vi "average_expSD.vi"(1 "Experiments groups":refnum<class "Experiments_group.lvclass">[](array[class]), 2 "group":u16) -> (0 "averaged data":dbl[][](array[numeric]))   [LabVIEW 2015]
uses:
  Classes/Experiment.lvclass
  Classes/Experiments_group.lvclass
panel:
  in  "error in (no error)":errorcluster
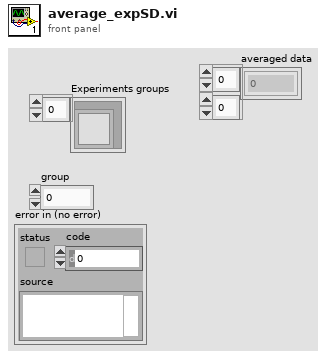
[diagram p1: front panel]
types:
  T1 = cluster{"Lower limit W":dbl, "Upper limit W":dbl}
  T2 = cluster{"Lower limit TD":dbl, "Upper limit TD":dbl}
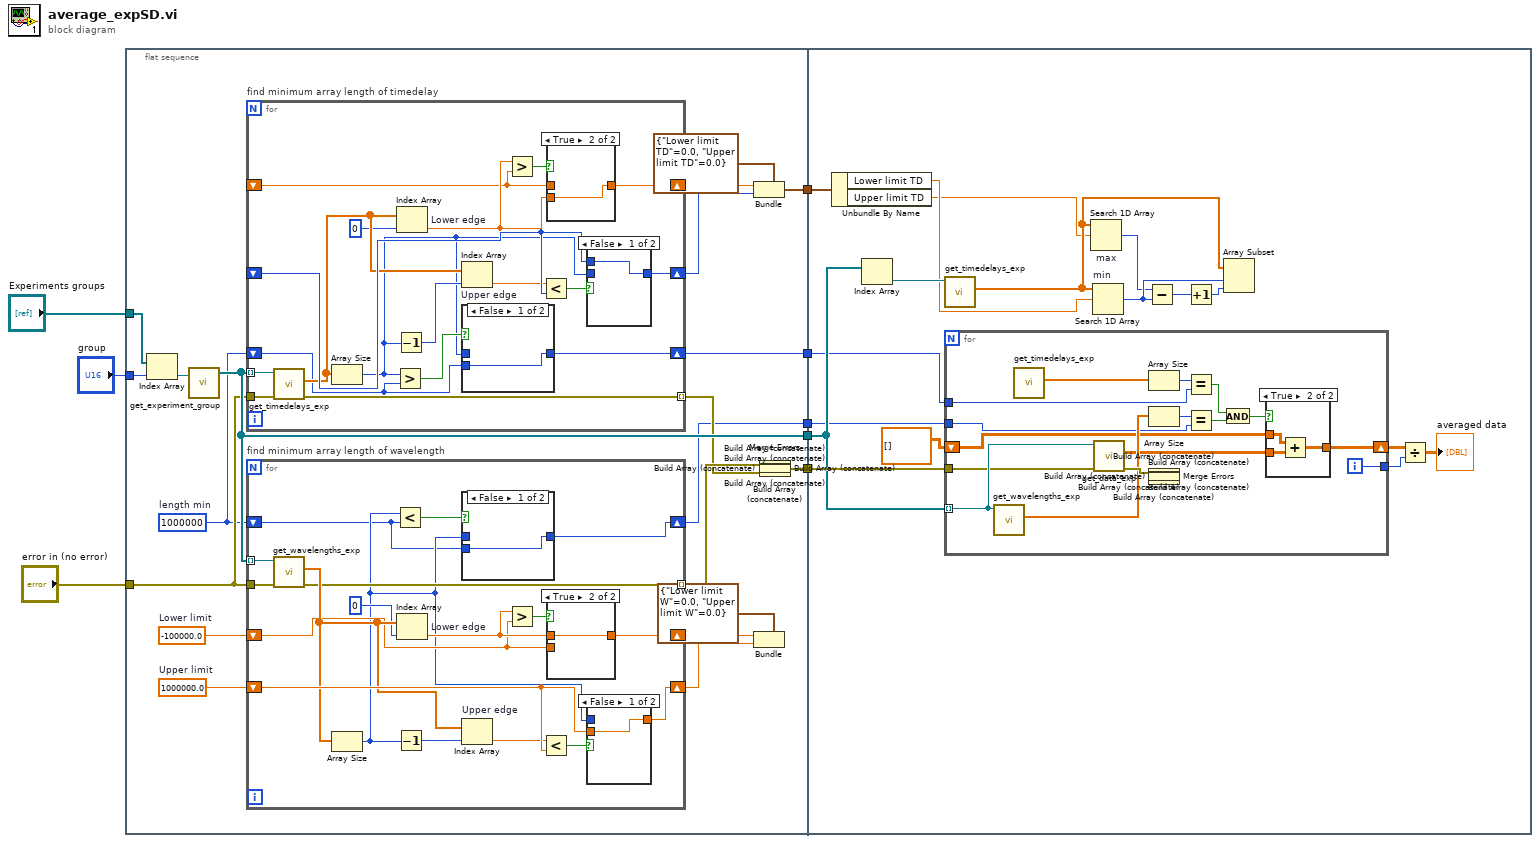
[diagram p0: block diagram]
diagram:
  n1 = flat-sequence {
    tunnel: "group" -> [w33]
    tunnel: "Experiments groups" -> [w32]
    tunnel: "error in (no error)" -> [w19]
    tunnel: [w23] -> w5
    tunnel: [w20] -> w4
    tunnel: [w18] -> w3
    tunnel: [w16] -> w2
    tunnel: [w15] -> w1
    tunnel: w5 -> [w88]
    tunnel: w4 -> [w95]
    tunnel: w3 -> [w94]
    tunnel: w2 -> [w84]
    tunnel: w1 -> [w83]
    frame #0 {
      w17 = 1000000  # length min
      w30 = -100000.0  # Lower limit
      w31 = 1000000.0  # Upper limit
      n2 = Index Array(array=w32, index=w33) -> (element=w34:refnum<class "Experiments_group.lvclass">)
      n3 = call-dynamic "get_experiment_group.vi"("Experiments_group.lvclass in"=w34) -> ("Experiments"=w23:refnum<class "Experiment.lvclass">[])  [unwired: 1 in, 2 out]
      n4 = for "find minimum array length of timedelay" {
        tunnel: w23 -> [w52] mode=indexing
        tunnel: w19 -> [w51]
        shift-right: [w49] -> w25
        shift-left: _ -> [w48]
        shift-right: [w42] -> w24
        shift-left: _ -> [w41]
        tunnel: [w39] -> w21 mode=indexing
        shift-right: [w37] -> w15
        shift-left: w17 -> [w35]
        n5 = call-dynamic "get_timedelays_exp.vi"("error in (no error)"=w51, "Experiment.lvclass in"=w52) -> ("error out"=w39:errorcluster, "timedelays"=w45:dbl[])  [unwired: 7 in, 1 out]
        n6 = Array Size(array=w45) -> (size(s)=w36:i32)
        n7 = Greater?(x=w36, y=w35) -> (0:w38:bool)
        n8 = Decrement(x=w36) -> (x-1=w47:i32)
        n9 = Index Array "Lower edge"(array=w45, index=0) -> (element=w43:dbl)
        n10 = Index Array "Upper edge"(array=w45, index=w47) -> (element=w46:dbl)
        n11 = case shown="False" w38 {
          tunnel: [w53 w54] -> w37
          tunnel: w36 -> [_ w54]
          tunnel: w35 -> [w53 _]
          frame False {
          }
          frame True {
          }
        }
        n12 = Greater?(x=w43, y=w41) -> (0:w40:bool)
        n13 = Less?(x=w46, y=w48) -> (x < y?=w50:bool)
        n14 = case shown="True" w40 {
          tunnel: [w55 w56] -> w42
          tunnel: w43 -> [_ w56]
          tunnel: w41 -> [w55 _]
          frame False {
          }
          frame True {
          }
        }
        n15 = case shown="False" w50 {
          tunnel: [w57 w58] -> w49
          tunnel: w36 -> [_ w58]
          tunnel: w48 -> [w57 _]
          frame False {
          }
          frame True {
          }
        }
      }
      n16 = for "find minimum array length of wavelength" {
        tunnel: w23 -> [w76] mode=indexing
        tunnel: w19 -> [w75]
        shift-right: [w73] -> w28
        shift-left: w31 -> [w72]
        shift-right: [w66] -> w29
        shift-left: w30 -> [w65]
        tunnel: [w63] -> w22 mode=indexing
        shift-right: [w60] -> w16
        shift-left: w17 -> [w59]
        n17 = call-dynamic "get_wavelengths_exp.vi"("error in (no error)"=w75, "Experiment.lvclass in"=w76) -> ("error out"=w63:errorcluster, "wavelengths"=w69:dbl[])  [unwired: 7 in, 1 out]
        n18 = Array Size(array=w69) -> (size(s)=w61:i32)
        n19 = Less?(x=w61, y=w59) -> (x < y?=w62:bool)
        n20 = Decrement(x=w61) -> (x-1=w71:i32)
        n21 = Index Array "Lower edge"(array=w69, index=0) -> (element=w67:dbl)
        n22 = case shown="False" w62 {
          tunnel: w61 -> [_ w78]
          tunnel: [w77 w78] -> w60
          tunnel: w59 -> [w77 _]
          frame False {
          }
          frame True {
          }
        }
        n23 = Index Array "Upper edge"(array=w69, index=w71) -> (element=w70:dbl)
        n24 = Greater?(x=w67, y=w65) -> (0:w64:bool)
        n25 = Less?(x=w70, y=w72) -> (x < y?=w74:bool)
        n26 = case shown="True" w64 {
          tunnel: [w79 w80] -> w66
          tunnel: w67 -> [_ w80]
          tunnel: w65 -> [w79 _]
          frame False {
          }
          frame True {
          }
        }
        n27 = case shown="False" w74 {
          tunnel: [w81 w82] -> w73
          tunnel: w61 -> [_ w82]
          tunnel: w72 -> [w81 _]
          frame False {
          }
          frame True {
          }
        }
      }
      n28 = Bundle(cluster=T2 {"Lower limit TD"=0.0, "Upper limit TD"=0.0}, "Lower limit TD"=w24, "Upper limit TD"=w25) -> (w18:T2)
      n29 = Bundle(cluster=T1 {"Lower limit W"=0.0, "Upper limit W"=0.0}, "Lower limit W"=w29, "Upper limit W"=w28) -> ()  [unwired: 1 out]
      n30 = Build Array (concatenate)(w22, w21) -> (w14:errorcluster[])
      n31 = Build Array (concatenate)(w14) -> (w13:errorcluster[])
      n32 = Build Array (concatenate)(w13) -> (w12:errorcluster[])
      n33 = Build Array (concatenate)(w12) -> (w11:errorcluster[])
      n34 = Build Array (concatenate)(w11) -> (w10:errorcluster[])
      n35 = Build Array (concatenate)(w10) -> (w9:errorcluster[])
      n36 = Merge Errors(w9) -> (w20:errorcluster)
    }
    frame #1 {
      n37 = Unbundle By Name(w94) -> ("Lower limit TD"=w86:dbl, "Upper limit TD"=w85:dbl)
      n38 = Index Array(array=w88) -> (element=w87:refnum<class "Experiment.lvclass">)  [unwired: 1 in]
      n39 = call-dynamic "get_timedelays_exp.vi"("Experiment.lvclass in"=w87) -> ("timedelays"=w89:dbl[])  [unwired: 8 in, 2 out]
      n40 = for {
        tunnel: w88 -> [w121] mode=indexing
        shift-right: [w106] -> w97
        shift-left: dbl[][] [] ("Data") -> [w108]
        tunnel: w95 -> [w118]
        tunnel: w84 -> [w113]
        tunnel: w83 -> [w112]
        tunnel: [w122] -> w98
        i -> [w122]
        n41 = call-dynamic "get_wavelengths_exp.vi"("Experiment.lvclass in"=w121) -> ("error out"=w120:errorcluster, "wavelengths"=w117:dbl[])  [unwired: 8 in, 1 out]
        n42 = call-dynamic "get_timedelays_exp.vi"() -> ("timedelays"=w116:dbl[])  [unwired: 9 in, 2 out]
        n43 = call-dynamic "get_data_exp.vi"("error in (no error)"=w118, "Experiment.lvclass in"=w121) -> ("error out"=w119:errorcluster, "Data"=w107:dbl[][])  [unwired: 7 in, 1 out]
        n44 = Array Size(array=w116) -> (size(s)=w115:i32)
        n45 = Array Size(array=w117) -> (size(s)=w114:i32)
        n46 = Build Array (concatenate)(w119) -> (w105:errorcluster[])  [unwired: 1 in]
        n47 = Build Array (concatenate)(w105) -> (w104:errorcluster[])
        n48 = Build Array (concatenate)(w104) -> (w103:errorcluster[])
        n49 = Build Array (concatenate)(w103) -> (w102:errorcluster[])
        n50 = Build Array (concatenate)(w102) -> (w101:errorcluster[])
        n51 = Build Array (concatenate)(w101) -> (w100:errorcluster[])
        n52 = Merge Errors(w100) -> ()  [unwired: 1 out]
        n53 = Equal?(x=w115, y=w112) -> (x = y?=w111:bool)
        n54 = Equal?(x=w114, y=w113) -> (x = y?=w110:bool)
        n55 = And(x=w111, y=w110) -> (x .and. y?=w109:bool)
        n56 = case shown="True" w109 {
          tunnel: w108 -> [_ w125]
          tunnel: w107 -> [_ w124]
          tunnel: [_ w123] -> w106
          frame False {
          }
          frame True {
            n57 = Add(x=w125, y=w124) -> (x+y=w123:dbl[][])
          }
        }
      }
      n58 = Search 1D Array "max"(1D array=w89, element=w85) -> (index of element=w90:i32)  [unwired: 1 in]
      n59 = Search 1D Array "min"(1D array=w89, element=w86) -> (index of element=w91:i32)  [unwired: 1 in]
      n60 = Subtract(x=w90, y=w91) -> (x-y=w92:i32)
      n61 = Increment(x=w92) -> (x+1=w93:i32)
      n62 = Array Subset(array=w89, index=w91, length=w93) -> ()  [unwired: 1 out]
      n63 = Divide(x=w97, y=w98) -> (x/y=→"averaged data":dbl[][])
    }
  }
